vi "IsStepLessThenSize.vi"(10 "all rows":i64[][](array[numeric]), 11 "Current step":i32) -> (3 "Boolean":bool)   [LabVIEW 2017]
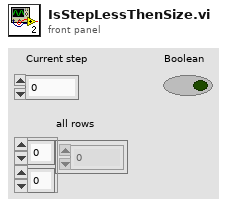
[diagram p1: front panel]
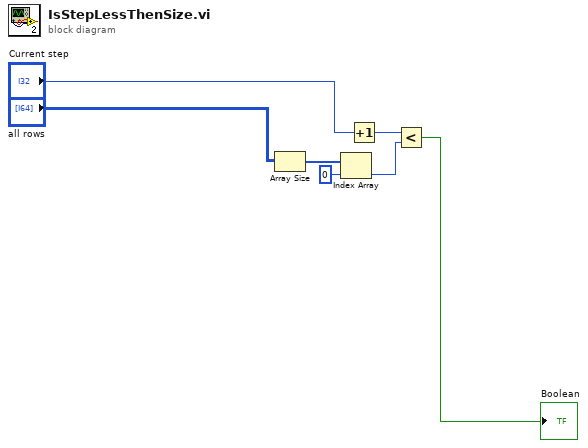
[diagram p0: block diagram]
diagram:
  n1 = Array Size(array="all rows") -> (size(s)=w2:i32[])
  n2 = Index Array(array=w2, index=0) -> (element=w4:i32)
  n3 = Increment(x="Current step") -> (x+1=w5:i32)
  n4 = Less?(x=w5, y=w4) -> (x < y?=→"Boolean":bool)
